vi "Filter Classes By Parent.vi"(7 "Parent Class":refnum<class>, 8 "error in (no error)":errorcluster, 10 "Class References":refnum<vi>[](array[refnum])) -> (0 "error out":errorcluster, 2 "Class References":refnum<vi>[](array[refnum]))   [LabVIEW 2020, in "Process Generation.lvlib" / "New Class Dialog.lvclass"]
uses:
  New Class Dialog.lvclass
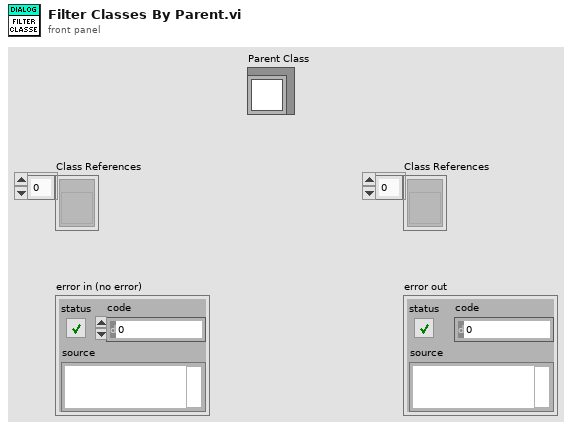
[diagram p1: front panel]
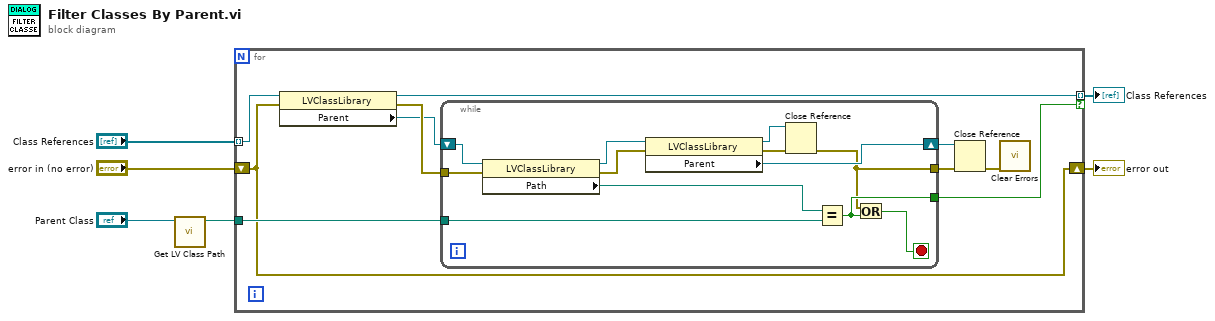
[diagram p0: block diagram]
diagram:
  n1 = call <vilib>:"Get LV Class Path.vi"("object"="Parent Class") -> ("class path"=w4:path)  [unwired: 9 in, 1 out]
  n2 = for {
    tunnel: "Class References" -> [w11] mode=indexing
    shift-right: [w9] -> w2
    shift-left: "error in (no error)" -> [w9]
    tunnel: [w12] -> w1 mode=indexing if=w16
    tunnel: w4 -> [w15]
    n3 = property class="LVClassLibrary"(reference=w11, error in=w9) -> (reference out=w12:refnum<vi>, error out=w14:errorcluster, "Parent"=w13:refnum<vi>)
    n4 = while {
      tunnel: [w26] -> w16
      shift-right: [w20] -> w10
      shift-left: w13 -> [w23]
      tunnel: w15 -> [w25]
      tunnel: w14 -> [w24]
      tunnel: [w17] -> w8
      stop <- w27 stop-if-true
      n5 = property class="LVClassLibrary"(reference=w23, error in=w24) -> (reference out=w21:refnum<vi>, error out=w22:errorcluster, "Path"=w28:path)
      n6 = property class="LVClassLibrary"(reference=w21, error in=w22) -> (reference out=w18:refnum<vi>, error out=w19:errorcluster, "Parent"=w20:refnum<vi>)
      n7 = Close Reference(reference=w18, error in (no error)=w19) -> (error out=w17:errorcluster)
      n8 = Equal?(x=w28, y=w25) -> (x = y?=w26:bool)
      n9 = Or(x=w17, y=w26) -> (x .or. y?=w27:bool)
    }
    n10 = Close Reference(reference=w10, error in (no error)=w8) -> (error out=w7:errorcluster)
    n11 = call <vilib>:"Clear Errors.vi"("error in (no error)"=w7) -> ()  [unwired: 5 in, 2 out]
  }
  "error out" <- w2
  "Class References" <- w1
